vi "Get Correct Target.vi"(1 "4":bool, 2 "2":bool, 3 "3":bool, 4 "Target Info":T2(array[cluster]), 5 "Target Found?":bool, 6 "1":bool) -> (0 "Selected Target Info":T1)   [LabVIEW 2012]
panel:
  out "appended array":dbl[](array[numeric])
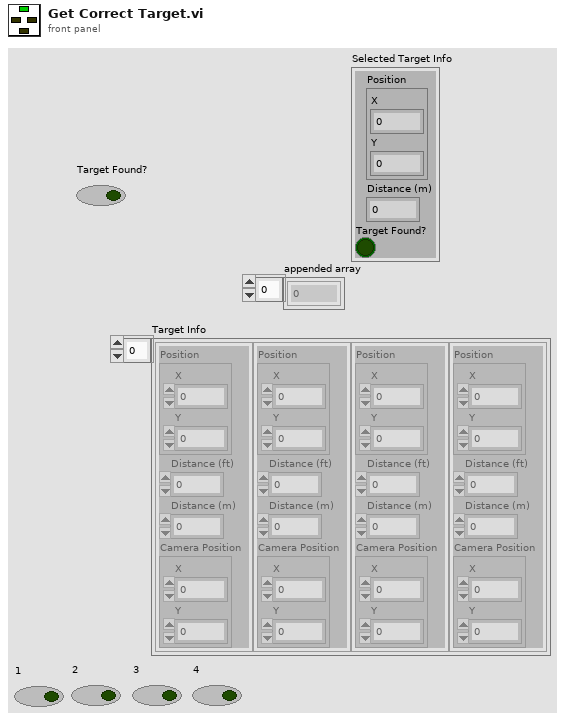
[diagram p1: front panel]
types:
  T1 = cluster{"Position":cluster{"X":dbl, "Y":dbl}, "Distance (m)":dbl, "Target Found?":bool}
  T2 = cluster{"Position":cluster{"X":dbl, "Y":dbl}, "Distance (ft)":dbl, "Distance (m)":dbl, "Camera Position":cluster{"X":dbl, "Y":dbl}}[]
  T3 = cluster{"Target Info[0]":cluster{"Position":cluster{"X":dbl, "Y":dbl}, "Distance (ft)":dbl, "Distance (m)":dbl, "Camera Position":cluster{"X":dbl, "Y":dbl}}, "Target Info[1]":cluster{"Position":cluster{"X":dbl, "Y":dbl}, "Distance (ft)":dbl, "Distance (m)":dbl, "Camera Position":cluster{"X":dbl, "Y":dbl}}, "Target Info[2]":cluster{"Position":cluster{"X":dbl, "Y":dbl}, "Distance (ft)":dbl, "Distance (m)":dbl, "Camera Position":cluster{"X":dbl, "Y":dbl}}, "Target Info[3]":cluster{"Position":cluster{"X":dbl, "Y":dbl}, "Distance (ft)":dbl, "Distance (m)":dbl, "Camera Position":cluster{"X":dbl, "Y":dbl}}, "Target Info[4]":cluster{"Position":cluster{"X":dbl, "Y":dbl}, "Distance (ft)":dbl, "Distance (m)":dbl, "Camera Position":cluster{"X":dbl, "Y":dbl}}, "Target Info[5]":cluster{"Position":cluster{"X":dbl, "Y":dbl}, "Distance (ft)":dbl, "Distance (m)":dbl, "Camera Position":cluster{"X":dbl, "Y":dbl}}, "Target Info[6]":cluster{"Position":cluster{"X":dbl, "Y":dbl}, "Distance (ft)":dbl, "Distance (m)":dbl, "Camera Position":cluster{"X":dbl, "Y":dbl}}, "Target Info[7]":cluster{"Position":cluster{"X":dbl, "Y":dbl}, "Distance (ft)":dbl, "Distance (m)":dbl, "Camera Position":cluster{"X":dbl, "Y":dbl}}, "Target Info[8]":cluster{"Position":cluster{"X":dbl, "Y":dbl}, "Distance (ft)":dbl, "Distance (m)":dbl, "Camera Position":cluster{"X":dbl, "Y":dbl}}}
  T4 = cluster{"Position":cluster{"X":dbl, "Y":dbl}, "Distance (ft)":dbl, "Distance (m)":dbl, "Camera Position":cluster{"X":dbl, "Y":dbl}}
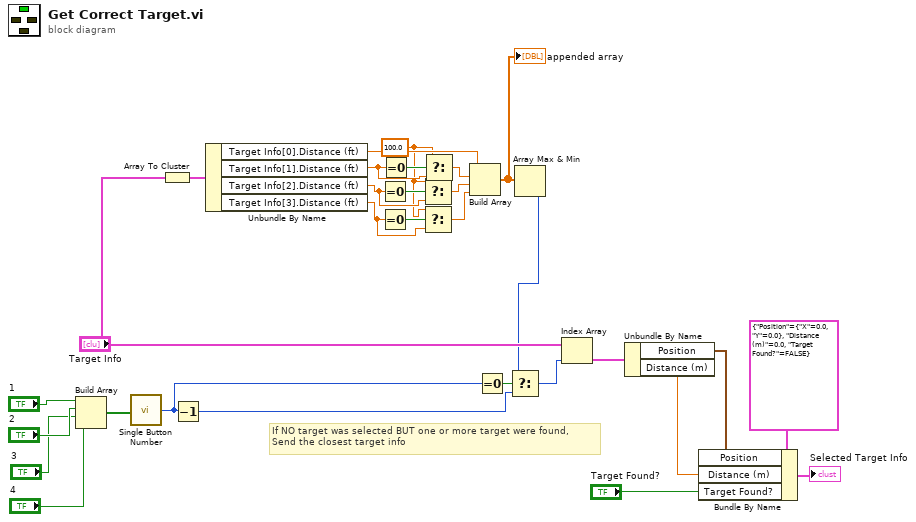
[diagram p0: block diagram]
diagram:
  w4 = 100.0 ("t")
  # "If NO target was selected BUT one or more target were found, \nSend the closest target info"
  n1 = Build Array("1", "2", "3", "4") -> (w26:bool[])
  n2 = call "Single Button Number.vi"("Bool Array"=w26) -> ("Number"=w14:i32)
  n3 = Array To Cluster(array="Target Info") -> (cluster=w18:T3)
  n4 = Decrement(x=w14) -> (x-1=w12:i32)
  n5 = Unbundle By Name(w18) -> ("Target Info[0].Distance (ft)"=w17:dbl, "Target Info[1].Distance (ft)"=w5:dbl, "Target Info[2].Distance (ft)"=w6:dbl, "Target Info[3].Distance (ft)"=w7:dbl)
  n6 = Equal To 0?(x=w6) -> (x = 0?=w9:bool)
  n7 = Equal To 0?(x=w7) -> (x = 0?=w8:bool)
  n8 = Equal To 0?(x=w5) -> (x = 0?=w10:bool)
  n9 = Select(t=w4, s=w9, f=w6) -> (s? t:f=w2:dbl)
  n10 = Select(t=w4, s=w8, f=w7) -> (s? t:f=w1:dbl)
  n11 = Select(t=w4, s=w10, f=w5) -> (s? t:f=w3:dbl)
  n12 = Build Array(w17, w3, w2, w1) -> (w16:dbl[])
  "appended array" <- w16
  n13 = Equal To 0?(x=w14) -> (x = 0?=w15:bool)
  n14 = Array Max & Min(array=w16) -> (min index (indices)=w13:i32)  [unwired: 3 out]
  n15 = Select(t=w13, s=w15, f=w12) -> (s? t:f=w11:i32)
  n16 = Index Array(array="Target Info", index=w11) -> (element=w25:T4)
  n17 = Unbundle By Name(w25) -> ("Position"=w24:cluster{"X":dbl, "Y":dbl}, "Distance (m)"=w23:dbl)
  n18 = Bundle By Name(cluster=T1 {"Position"={"X"=0.0, "Y"=0.0}, "Distance (m)"=0.0, "Target Found?"=FALSE} ("input cluster"), "Position"=w24, "Distance (m)"=w23, "Target Found?"="Target Found?") -> (→"Selected Target Info":T1)
